vi "Set_Current_Range.vi"(5 "Current Range Ch 2":T1 items=["Autorange", "+/- 20 mikroA", "+/- 2 mikroA", "+/- 200 nA", "+/- 20 nA", "+/- 2 nA"], 6 "GPIB (t) / RS-232 (f)":bool, 7 "Current Range Ch 1":T1 items=["Autorange", "+/- 20 mikroA", "+/- 2 mikroA", "+/- 200 nA", "+/- 20 nA", "+/- 2 nA"], 8 "error in (no error)":errorcluster, 11 "VISA resource name":refnum<visa-resource-name>) -> (0 "error out":errorcluster, 3 "VISA resource name out":refnum<visa-resource-name>)   [LabVIEW 2018]
uses:
  Current_Range_Control.ctl
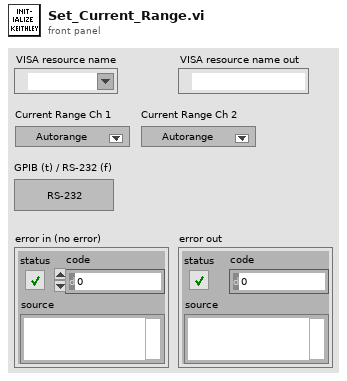
[diagram p1: front panel]
types:
  T1 = typedef "Current_Range_Control.ctl" = u16
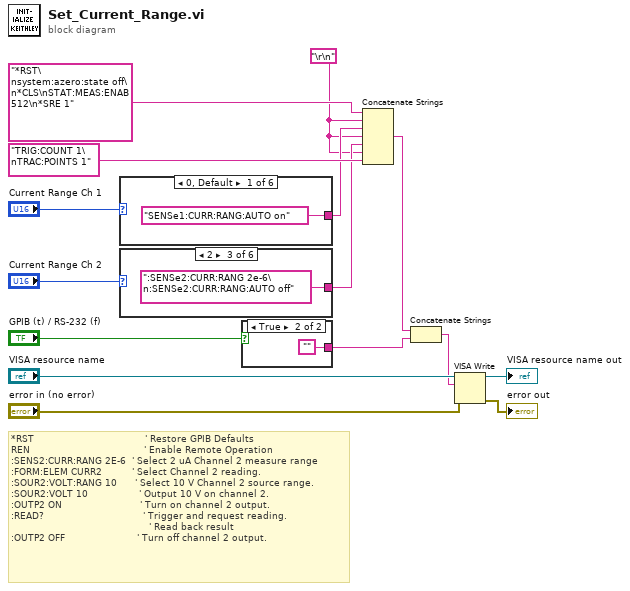
[diagram p0: block diagram]
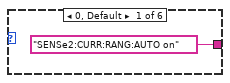
[diagram p2: hidden frame]
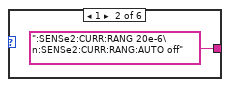
[diagram p3: hidden frame]
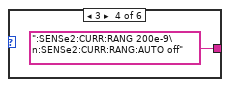
[diagram p4: hidden frame]
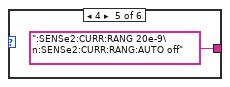
[diagram p5: hidden frame]
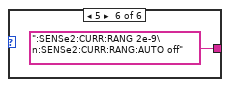
[diagram p6: hidden frame]
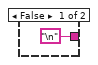
[diagram p7: hidden frame]
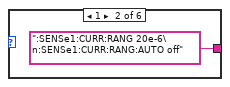
[diagram p8: hidden frame]
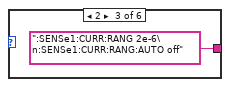
[diagram p9: hidden frame]
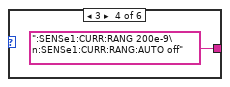
[diagram p10: hidden frame]
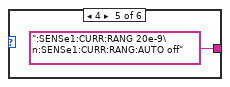
[diagram p11: hidden frame]
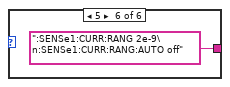
[diagram p12: hidden frame]
diagram:
  w1 = "\r\n"
  # "*RST \t\t\t                                 ' Restore GPIB Defaults\nREN                                      ' Enable Remote Operation\n:SENS2:CURR:RANG 2E-6 \t' Select 2 uA Channel 2 measure range\n:FORM:ELEM CURR2 \t        ' Select Channel 2 reading.\n:SOUR2:VOLT:RANG 10 \t    ' Select 10 V Channel 2 source range.\n:SOUR2:VOLT 10 \t\t              ' Output 10 V on channel 2.\n:OUTP2 ON \t\t                       ' Turn on channel 2 output.\n:READ? \t\t\t                             ' Trigger and request reading.\n\t\t\t                                           ' Read back result\n:OUTP2 OFF \t\t                     ' Turn off channel 2 output."
  n1 = case shown="0, Default" "Current Range Ch 1" {
    tunnel: ["SENSe1:CURR:RANG:AUTO on" ":SENSe1:CURR:RANG 20e-6\n:SENSe1:CURR:RANG:AUTO off" ":SENSe1:CURR:RANG 2e-6\n:SENSe1:CURR:RANG:AUTO off" ":SENSe1:CURR:RANG 200e-9\n:SENSe1:CURR:RANG:AUTO off" ":SENSe1:CURR:RANG 20e-9\n:SENSe1:CURR:RANG:AUTO off" ":SENSe1:CURR:RANG 2e-9\n:SENSe1:CURR:RANG:AUTO off"] -> w4
    frame 0, Default {
    }
    frame 1 {
    }
    frame 2 {
    }
    frame 3 {
    }
    frame 4 {
    }
    frame 5 {
    }
  }
  n2 = case shown="2" "Current Range Ch 2" {
    tunnel: ["SENSe2:CURR:RANG:AUTO on" ":SENSe2:CURR:RANG 20e-6\n:SENSe2:CURR:RANG:AUTO off" ":SENSe2:CURR:RANG 2e-6\n:SENSe2:CURR:RANG:AUTO off" ":SENSe2:CURR:RANG 200e-9\n:SENSe2:CURR:RANG:AUTO off" ":SENSe2:CURR:RANG 20e-9\n:SENSe2:CURR:RANG:AUTO off" ":SENSe2:CURR:RANG 2e-9\n:SENSe2:CURR:RANG:AUTO off"] -> w3
    frame 0, Default {
    }
    frame 1 {
    }
    frame 2 {
    }
    frame 3 {
    }
    frame 4 {
    }
    frame 5 {
    }
  }
  n3 = case shown="True" "GPIB (t) / RS-232 (f)" {
    tunnel: ["\n" ""] -> w8
    frame False {
    }
    frame True {
    }
  }
  n4 = Concatenate Strings("*RST\nsystem:azero:state off\n*CLS\nSTAT:MEAS:ENAB 512\n*SRE 1", w1, w4, w1, w3, w1, "TRIG:COUNT 1\nTRAC:POINTS 1") -> (w2:string)
  n5 = Concatenate Strings(w2, w8) -> (w10:string)
  n6 = VISA Write(VISA resource name="VISA resource name", write buffer=w10, error in (no error)="error in (no error)") -> (VISA resource name out=→"VISA resource name out":refnum<visa-resource-name>, error out=→"error out":errorcluster)  [unwired: 1 out]
